vi "参数选择.vi"(11 "项名":string[](array[string])) -> (3 "字符串":string)   [LabVIEW 2016, in "下拉列表.xctl"]
panel:
  in  "列表框":T1
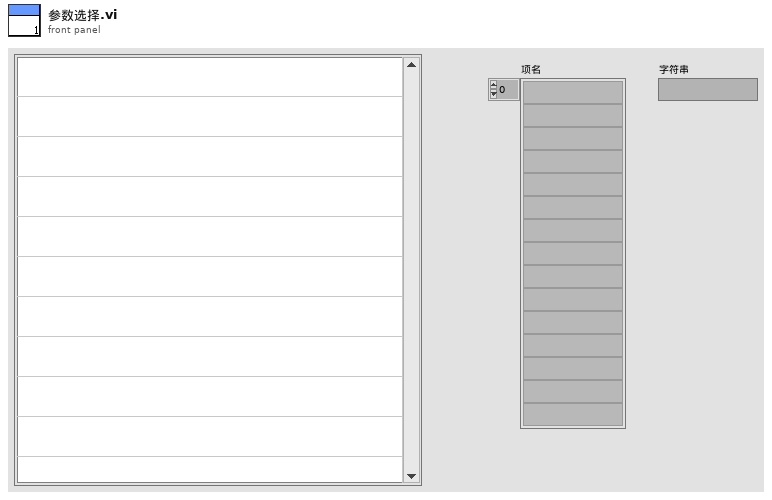
[diagram p1: front panel]
types:
  T1 = typedef "下拉列表.xctl/列表框.ctl" = i32
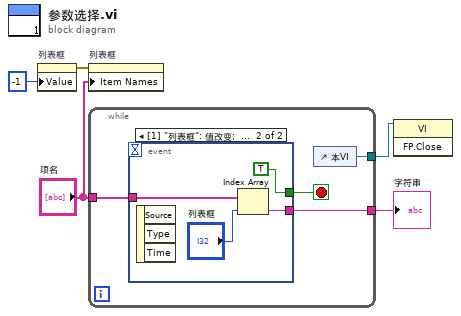
[diagram p0: block diagram]
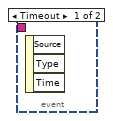
[diagram p2: hidden frame]
diagram:
  n1 = property on="列表框" class="LstBox (严格)"("Value"=T1 -1 ("列表框")) -> (error out=w3:errorcluster)  [unwired: 2 in, 1 out]
  n2 = property on="列表框" class="LstBox (严格)"(error in=w3, "Item Names"="项名") -> ()  [unwired: 1 in, 2 out]
  n3 = while {
    tunnel: "项名" -> [w9]
    tunnel: [w8] -> w4
    tunnel: [w6] -> w1
    stop <- w7 stop-if-true
    n4 = event shown="[1] \"列表框\": 值改变;  前面板关闭" {
      selector: _ -> [_ _]
      dyn-events: _ -> [_ _]
      timeout: _ -> [_ _]
      tunnel: w9 -> [_ w13]
      tunnel: [_ w11] -> w8
      tunnel: [_ TRUE] -> w7
      event Timeout {
        n5 = event-data() -> ()  [unwired: 1 in, 3 out]
      }
      event Value Change; Panel Close {
        n6 = event-data() -> ()  [unwired: 1 in, 3 out]
        n7 = Index Array(array=w13, index="列表框") -> (element=w11:string)
      }
    }
    n8 = control-ref of="本VI"() -> (w6:refnum<vi>)
  }
  "字符串" <- w4
  n9 = invoke class="VI" method="FP.Close"(reference=w1) -> ()  [unwired: 2 in, 3 out]
